vi "Update Matrix Config.vi"(8 "error in (no error)":errorcluster, 11 "Matrix Parameter":string[](array[string])) -> (0 "error out":errorcluster, 3 "Matrix":T1={"Parameter"={"Ref"=variant, "topology name"="Configured Topology"}, "relay name"="k0", "relay action"=21, "First Connection"={"channel 1"="r0", "channel 2"="c0"}, "Second Connection"={"channel 3"="r1", "channel 4"="c1"}} {"relay action" items=["Open Relay"=20, "Close Relay"=21]})   [LabVIEW 2016, in "S-Matrix.lvlib"]
uses:
  S-Matrix.lvlib
  Matrix Config Parameter.ctl
  Initialize Parameter.ctl
  User Interface/User Interface.lvlib
panel:
  in  "relay action":i32(ring)=21 items=["Open Relay"=20, "Close Relay"=21]
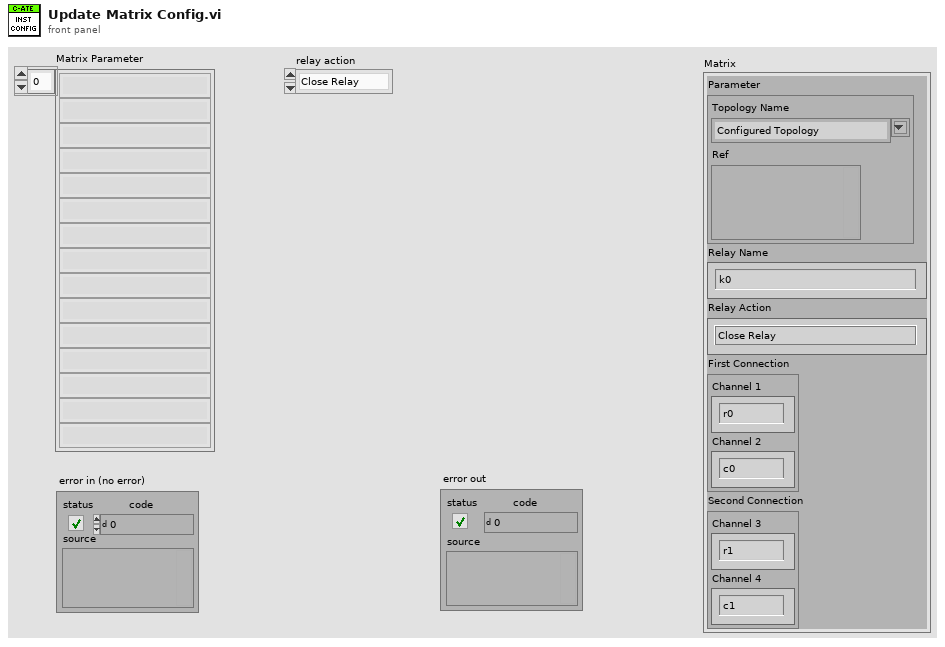
[diagram p1: front panel]
types:
  T1 = typedef "S-Matrix.lvlib/Matrix Config Parameter.ctl" = cluster{"Parameter":T2, "relay name":string, "relay action":i32, "First Connection":cluster{"channel 1":string, "channel 2":string}, "Second Connection":cluster{"channel 3":string, "channel 4":string}}
  T2 = typedef "S-Matrix.lvlib/Initialize Parameter.ctl" = cluster{"Ref":variant, "topology name":string}
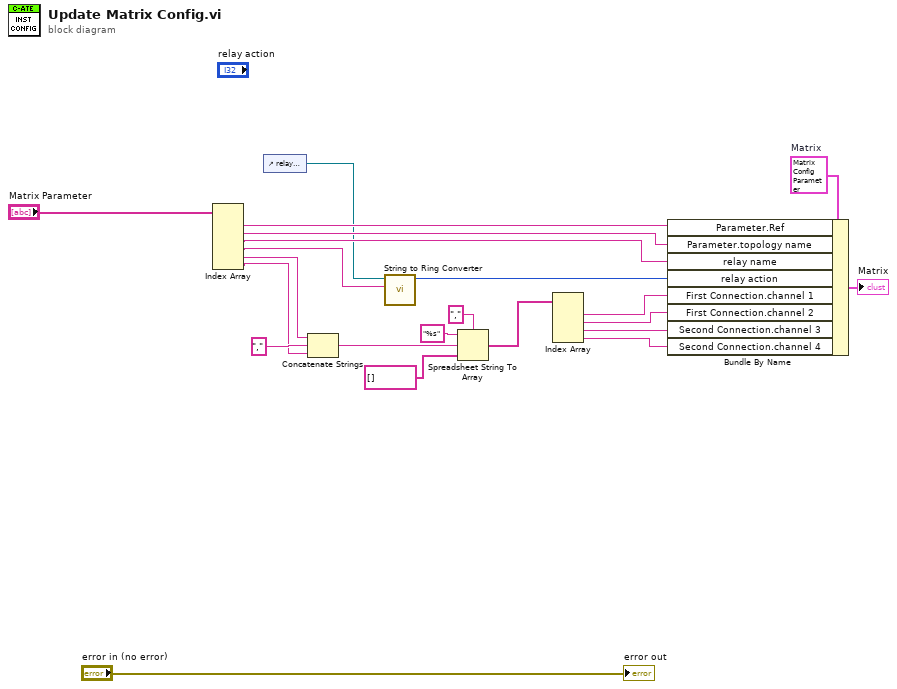
[diagram p0: block diagram]
diagram:
  w7 = T1 {"Parameter"={"Ref"=variant, "topology name"="Configured Topology"}, "relay name"="k0", "relay action"=21, "First Connection"={"channel 1"="r0", "channel 2"="c0"}, "Second Connection"={"channel 3"="r1", "channel 4"="c1"}}  # Matrix
  n1 = Index Array(array="Matrix Parameter") -> (element #1=w20:string, element #2=w19:string, element #3=w18:string, element #4=w16:string, element #5=w14:string, element #6=w11:string)  [unwired: 6 in]
  n2 = control-ref of="relay action"() -> (w17:refnum<vi>)
  n3 = Concatenate Strings(w14, "," ("string"), w11) -> (w8:string)
  n4 = call "String to Ring Converter.vi"("Control Name"=w16, "Ring Control"=w17) -> ("Value"=w15:i32)  [unwired: 9 in]
  n5 = Spreadsheet String To Array(delimiter (Tab)=",", format string="%s", spreadsheet string=w8, array type (2D Dbl)=string[] []) -> (array=w6:string[])
  n6 = Index Array(array=w6) -> (element #1=w5:string, element #2=w4:string, element #3=w3:string, element #4=w2:string)  [unwired: 4 in]
  n7 = Bundle By Name(cluster=w7, "Parameter.Ref"=w20, "Parameter.topology name"=w19, "relay name"=w18, "relay action"=w15, "First Connection.channel 1"=w5, "First Connection.channel 2"=w4, "Second Connection.channel 3"=w3, "Second Connection.channel 4"=w2) -> (→"Matrix":T1)
  "error out" <- "error in (no error)"
